vi "TempSensorDataCollection.vi"() -> ()   [LabVIEW 2023]
panel:
  in  "Select sensor":u16(ring) items=["T.A.101.2", "T.A.204.1", "T.A.301.1"]
  out "Temperature Sensor T.A.204.1":dbl(graph)
  in  "stop":bool
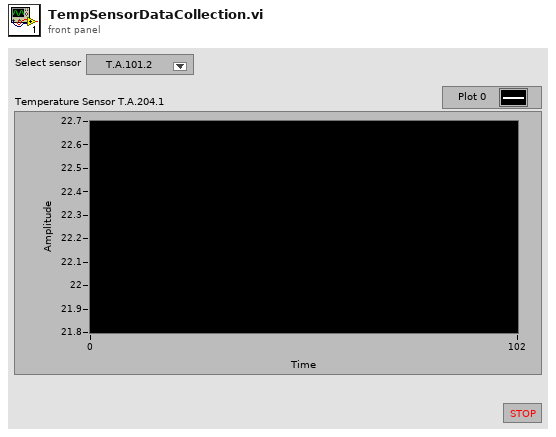
[diagram p1: front panel]
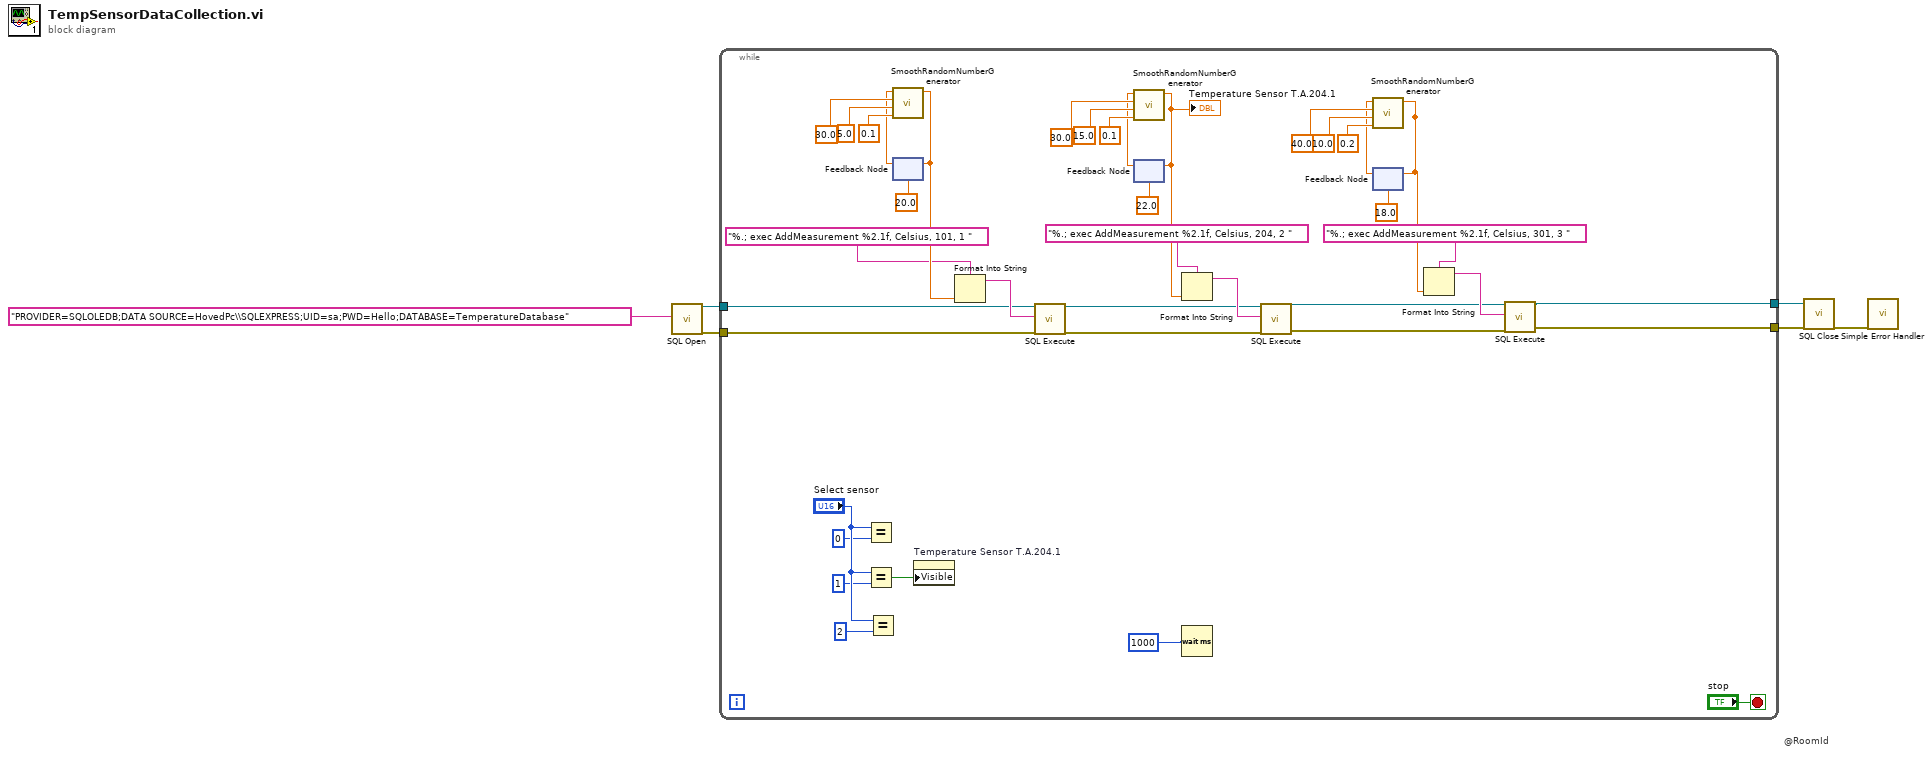
[diagram p0: block diagram]
diagram:
  # "@RoomId"
  n1 = call "SQL Open.vi"("ConnectionString In"="PROVIDER=SQLOLEDB;DATA SOURCE=HovedPc\\SQLEXPRESS;UID=sa;PWD=Hello;DATABASE=TemperatureDatabase") -> ("Connection Out"=w5:refnum<k7>, "Error out"=w4:errorcluster)  [unwired: 17 in]
  n2 = while {
    tunnel: w5 -> [w21]
    tunnel: w4 -> [w20]
    tunnel: [w11] -> w3
    tunnel: [w10] -> w2
    stop <- "stop" stop-if-true
    n3 = Equal?(x="Select sensor", y=u16 0) -> (x = y?=w35:bool)
    n4 = Equal?(x="Select sensor", y=u16 1) -> (x = y?=w24:bool)
    n5 = Equal?(x="Select sensor", y=u16 2) -> (x = y?=w34:bool)
    n6 = feedback #1(20.0 ("New val")) -> (w44:dbl)
    n7 = call "SmoothRandomNumberGenerator.vi"("Max step size"=0.1, "Bottom range"=5.0, "Top range"=30.0, "Old val"=w44) -> ("New val"=w22:dbl)  [unwired: 7 in]
    n8 = feedback-in #1(w22) -> ()
    n9 = property on="Temperature Sensor T.A.204.1" class="WFChart (strict)"("Visible"=w24) -> ()  [unwired: 2 in, 2 out]
    n10 = Format Into String(format string="%.; exec AddMeasurement %2.1f, Celsius, 101, 1 ", w22) -> (resulting string=w23:string)  [unwired: 2 in, 1 out]
    n11 = call "SQL Execute.vi"("Connection In"=w21, "SQL Query"=w23, "Error in (no error)"=w20) -> ("Connection Out"=w17:refnum<k7>, "Error out"=w16:errorcluster)  [unwired: 15 in]
    n12 = feedback #2(22.0 ("New val")) -> (w37:dbl)
    n13 = call "SmoothRandomNumberGenerator.vi"("Max step size"=0.1, "Bottom range"=15.0, "Top range"=30.0, "Old val"=w37) -> ("New val"=w18:dbl)  [unwired: 7 in]
    "Temperature Sensor T.A.204.1" <- w18
    n14 = feedback-in #2(w18) -> ()
    n15 = Format Into String(format string="%.; exec AddMeasurement %2.1f, Celsius, 204, 2 ", w18) -> (resulting string=w19:string)  [unwired: 2 in, 1 out]
    n16 = Wait (ms)(milliseconds to wait=u32 1000) -> ()  [unwired: 1 out]
    n17 = call "SQL Execute.vi"("Connection In"=w17, "SQL Query"=w19, "Error in (no error)"=w16) -> ("Connection Out"=w13:refnum<k7>, "Error out"=w12:errorcluster)  [unwired: 15 in]
    n18 = feedback #3(18.0 ("New val")) -> (w26:dbl)
    n19 = call "SmoothRandomNumberGenerator.vi"("Max step size"=0.2, "Bottom range"=10.0, "Top range"=40.0, "Old val"=w26) -> ("New val"=w14:dbl)  [unwired: 7 in]
    n20 = feedback-in #3(w14) -> ()
    n21 = Format Into String(format string="%.; exec AddMeasurement %2.1f, Celsius, 301, 3 ", w14) -> (resulting string=w15:string)  [unwired: 2 in, 1 out]
    n22 = call "SQL Execute.vi"("Connection In"=w13, "SQL Query"=w15, "Error in (no error)"=w12) -> ("Connection Out"=w11:refnum<k7>, "Error out"=w10:errorcluster)  [unwired: 15 in]
  }
  n23 = call "SQL Close.vi"("Connection In"=w3, "Error in (no error)"=w2) -> ("Error out"=w1:errorcluster)  [unwired: 17 in]
  n24 = call <vilib>:"Simple Error Handler.vi"("error in (no error)"=w1) -> ()  [unwired: 4 in, 5 out]
